vi "Description.vi"(8 "error in (no error)":errorcluster, 11 "Identical Inputs Comparator in":refnum<class "Identical Inputs Comparator.lvclass">) -> (0 "error out":errorcluster, 2 "Description":string)   [LabVIEW 2020, in "Identical Inputs Comparator.lvclass"]
uses:
  Identical Inputs Comparator.lvclass
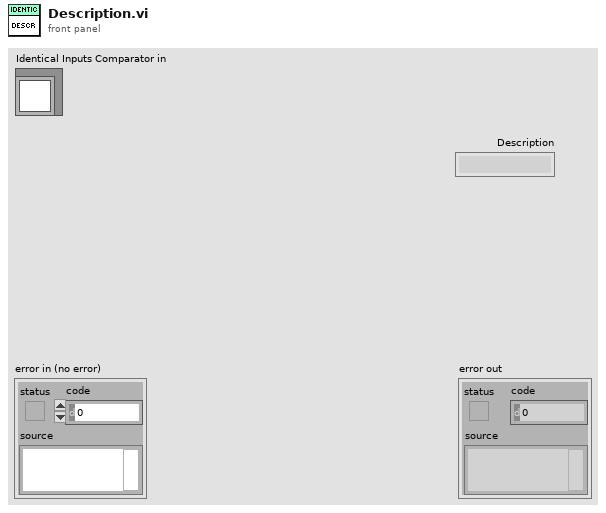
[diagram p1: front panel]
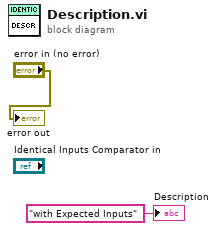
[diagram p0: block diagram]
diagram:
  "error out" <- "error in (no error)"
  "Description" <- "with Expected Inputs" ("Description")
